vi "SetUp.vi"(8 "error in (no error)":errorcluster, 11 "Prueba08 in":refnum<class "Prueba31.lvclass">) -> (0 "error out":errorcluster, 3 "Prueba08 out":refnum<class "Prueba31.lvclass">)   [LabVIEW 2019, in "Prueba31.lvclass"]
uses:
  Prueba31.lvclass
  Prueba31.lvclass/Prueba31.ctl
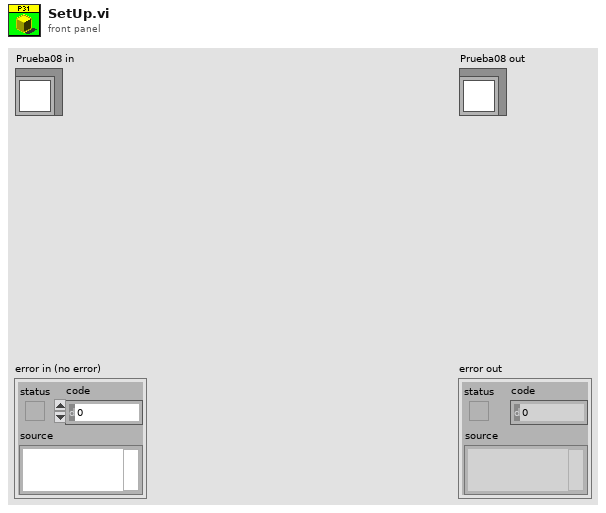
[diagram p1: front panel]
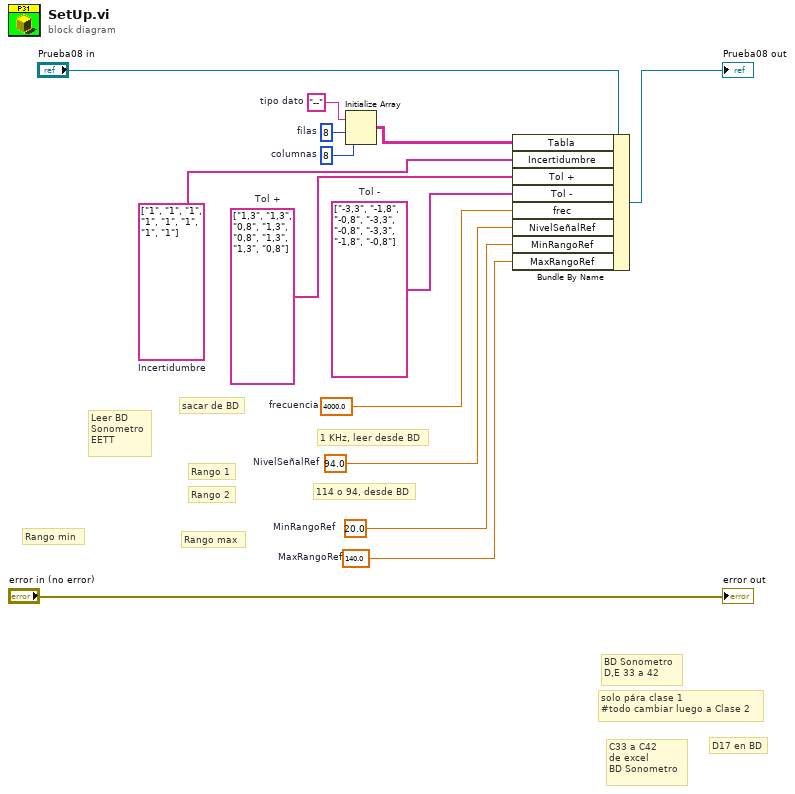
[diagram p0: block diagram]
diagram:
  w1 = 140.0  # MaxRangoRef
  w2 = 20.0  # MinRangoRef
  w13 = 94.0  # NivelSeñalRef
  w12 = 4000.0  # frecuencia
  w11 = string[] ["1", "1", "1", "1", "1", "1", "1", "1"]  # Incertidumbre
  w10 = string[] ["-3,3", "-1,8", "-0,8", "-3,3", "-0,8", "-3,3", "-1,8", "-0,8"]  # Tol -
  w9 = string[] ["1,3", "1,3", "0,8", "1,3", "0,8", "1,3", "1,3", "0,8"]  # Tol +
  w7 = 8  # columnas
  w6 = 8  # filas
  w8 = "--"  # tipo dato
  # "114 o 94, desde BD"
  # "1 KHz, leer desde BD"
  # "Rango 2"
  # "Rango 1"
  # "Rango max"
  # "Rango min"
  # "Leer BD\nSonometro\nEETT"
  # "sacar de BD"
  # "D17 en BD"
  # "BD Sonometro\nD,E 33 a 42"
  # "solo pára clase 1\n#todo cambiar luego a Clase 2"
  # "C33 a C42\nde excel\nBD Sonometro"
  n1 = Initialize Array(w8, w6, w7) -> (w5:string[][])
  n2 = Bundle By Name(cluster="Prueba08 in", "Tabla"=w5, "Incertidumbre"=w11, "Tol +"=w9, "Tol -"=w10, "frec"=w12, "NivelSeñalRef"=w13, "MinRangoRef"=w2, "MaxRangoRef"=w1) -> (→"Prueba08 out":refnum<class "Prueba31.lvclass">)
  "error out" <- "error in (no error)"
